vi "Export Configuration RTM.vi"(8 "error in (no error)":errorcluster, 11 "Node Ptr":u64 format="%.0x") -> (0 "error out":errorcluster)   [LabVIEW 2019, in "TemplatePPL System Explorer.lvlib"]
uses:
  TemplatePPL System Explorer.lvlib
  <vilib>/NI/NI VeriStand Custom Device Import and Export Tool/ImportExport.lvlib
panel:
  in  "Tag":string
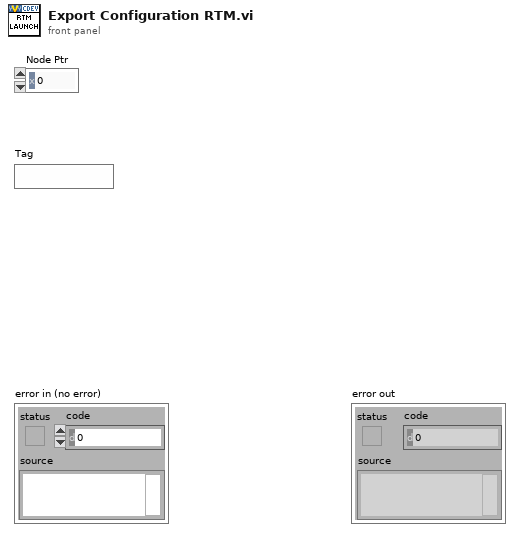
[diagram p1: front panel]
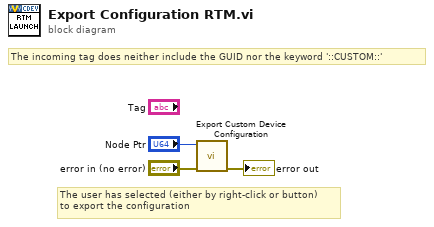
[diagram p0: block diagram]
diagram:
  # "The user has selected (either by right-click or button)\nto export the configuration"
  # "The incoming tag does neither include the GUID nor the keyword '::CUSTOM::'"
  n1 = call <vilib>:"Export Custom Device Configuration.vi"("error in (no error)"="error in (no error)", "ID"="Node Ptr") -> ("error out"=→"error out":errorcluster)  [unwired: 8 in, 1 out]
